vi "Parse Tasks.vi"(8 "error in (no error)":errorcluster, 11 "Tasks XML":string="<?xml version=\"1.0\" encoding=\"UTF-8\"?><ns2:instructions xmlns:ns2=\"http://jazz.net/xmlns/alm/qm/v0.1/\" xmlns:ns1=\"http://schema.ibm.com/vega/2008/\" xmlns:ns3=\"http://purl.org/dc/elements/1.1/\" xmlns:ns4=\"http://jazz.net/xmlns/prod/jazz/process/0.6/\" xmlns:ns5=\"http://jazz.net/xmlns/alm/v0.1/\" xmlns:ns6=\"http://www.w3.org/1999/02/22-rdf-syntax-ns#\" xmlns:ns7=\"http://purl.org/dc/terms/\" xmlns:ns8=\"http://jazz.net/xmlns/alm/qm/v0.1/tsl/v0.1/\" xmlns:ns9=\"http://jazz.net/xmlns/alm/qm/v0.1/testscript/v0.1/\" xmlns:ns10=\"http://jazz.net/xmlns/alm/qm/qmadapter/task/v0.1\" xmlns:ns11=\"http://jazz.net/xmlns/alm/qm/qmadapter/v0.1\" xmlns:ns12=\"http://jazz.net/xmlns/alm/qm/v0.1/executionworkitem/v0.1\" xmlns:ns13=\"http://jazz.net/xmlns/alm/qm/v0.1/executionresult/v0.1\" xmlns:ns14=\"http://jazz.net/xmlns/alm/qm/v0.1/catalog/v0.1\" xmlns:ns16=\"http://jazz.net/xmlns/alm/qm/styleinfo/v0.1/\" xmlns:ns17=\"http://www.w3.org/1999/XSL/Transform\"><ns11:workavailable>false</ns11:workavailable></ns2:instructions>") -> (0 "error out":errorcluster, 2 "First task URL":string)   [LabVIEW 2012]
uses:
  <vilib>/xml/Load XML String.vi
  <vilib>/xml/Close Reference(Node).vi
  <vilib>/xml/Close Reference(NNMap).vi
  <vilib>/xml/Close Reference(NdList).vi
  <vilib>/xml/NI_XML.lvlib
  <resource>/objmgr/DOMUserDefRef.rc
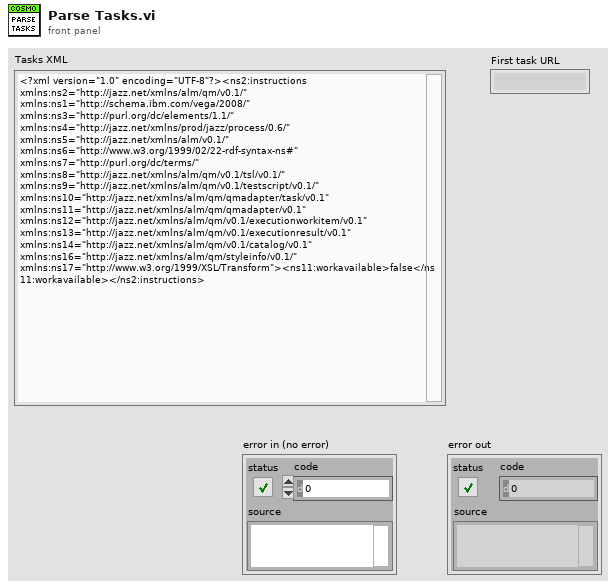
[diagram p1: front panel]
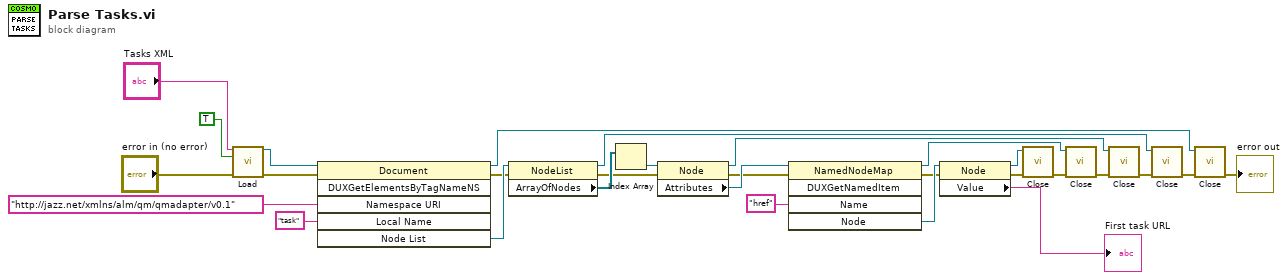
[diagram p0: block diagram]
diagram:
  n1 = call-poly <vilib>:"Load.vi"("XML string"="Tasks XML", "process namespaces (False)"=TRUE, "error in (no error)"="error in (no error)") -> ("DOM document out"=w22:refnum<k20>, "error out"=w24:errorcluster)  [unwired: 10 in, 1 out]
  n2 = invoke class="Document" method="DUXGetElementsByTagNameNS"(reference=w22, error in=w24, "Namespace URI"="http://jazz.net/xmlns/alm/qm/qmadapter/v0.1", "Local Name"="task") -> (reference out=w13:refnum<k20>, error out=w25:errorcluster, "Node List"=w26:refnum<k20>)  [unwired: 2 in, 3 out]
  n3 = property class="NodeList"(reference=w26, error in=w25) -> (reference out=w20:refnum<k20>, error out=w16:errorcluster, "ArrayOfNodes"=w23:refnum<k20>[])
  n4 = Index Array(array=w23) -> (element=w17:refnum<k20>)  [unwired: 1 in]
  n5 = property class="Node"(reference=w17, error in=w16) -> (reference out=w14:refnum<k20>, error out=w9:errorcluster, "Attributes"=w10:refnum<k20>)
  n6 = invoke class="NamedNodeMap" method="DUXGetNamedItem"(reference=w10, error in=w9, "Name"="href") -> (reference out=w4:refnum<k20>, error out=w6:errorcluster, "Node"=w7:refnum<k20>)  [unwired: 2 in, 2 out]
  n7 = property class="Node"(reference=w7, error in=w6) -> (reference out=w3:refnum<k20>, error out=w2:errorcluster, "Value"=→"First task URL":string)
  n8 = call-poly <vilib>:"Close.vi"("error in (no error)"=w2, "node"=w3) -> ("error out"=w5:errorcluster)  [unwired: 7 in]
  n9 = call-poly <vilib>:"Close.vi"("error in (no error)"=w5, "named node map"=w4) -> ("error out"=w11:errorcluster)  [unwired: 7 in]
  n10 = call-poly <vilib>:"Close.vi"("error in (no error)"=w11, "node"=w14) -> ("error out"=w19:errorcluster)  [unwired: 7 in]
  n11 = call-poly <vilib>:"Close.vi"("error in (no error)"=w19, "node list"=w20) -> ("error out"=w18:errorcluster)  [unwired: 7 in]
  n12 = call-poly <vilib>:"Close.vi"("error in (no error)"=w18, "node"=w13) -> ("error out"=→"error out":errorcluster)  [unwired: 7 in]
